vi "rqcSPI Write.vi"(9 "write data":bool, 11 "data in":u16) -> (1 "MOSI":bool, 2 "CLK":bool, 3 "CS":bool=TRUE)   [LabVIEW 2016]
uses:
  Custom Controls/rqcSPI Cluster.ctl
  Custom Controls/rqcSPI State.ctl
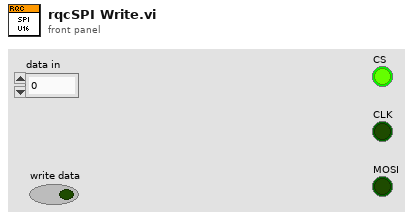
[diagram p1: front panel]
types:
  T1 = typedef "rqcSPI Cluster.ctl" = cluster{"state":T2, "bit's number":u8, "data":bool[], "CS":bool, "CLK":bool, "MOSI":bool}
  T2 = typedef "rqcSPI State.ctl" = enum16{"write", "idle"}
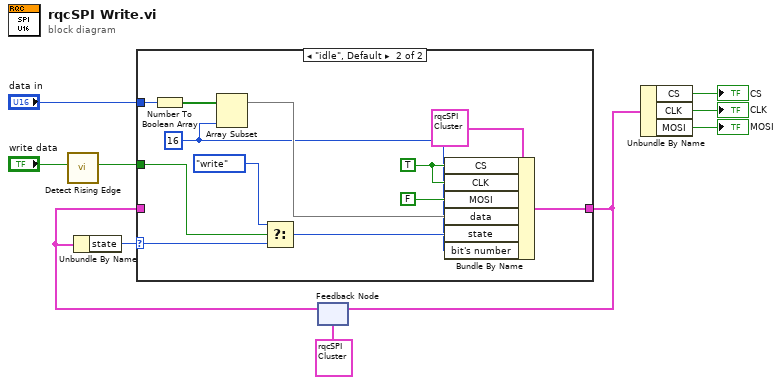
[diagram p0: block diagram]
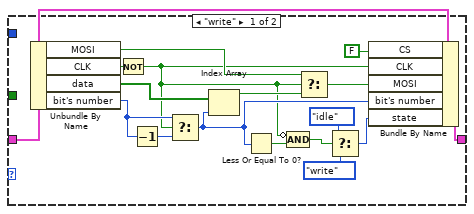
[diagram p2: hidden frame]
diagram:
  n1 = call <vilib>:"Detect Rising Edge.vi"("signal"="write data") -> ("edge detected"=w7:bool)  [unwired: 10 in]
  n2 = feedback #1(T1 {"state"=enum."idle", "bit's number"=16, "data"=[FALSE, FALSE, FALSE, FALSE, FALSE, FALSE, FALSE, FALSE, FALSE, FALSE, FALSE, FALSE, FALSE, FALSE, FALSE, FALSE], "CS"=TRUE, "CLK"=TRUE, "MOSI"=FALSE} ("rqcSPI Cluster")) -> (w6:T1)
  n3 = Unbundle By Name(w6) -> ("state"=w9:T2)
  n4 = case shown="\"idle\", Default" w9 {
    selector: w9 -> [_ w35]
    tunnel: w7 -> [_ w37]
    tunnel: w6 -> [w27 _]
    tunnel: "data in" -> [_ w38]
    tunnel: [w26 w33] -> w4
    frame "write" {
      n5 = Unbundle By Name(w27) -> ("MOSI"=w22:bool, "CLK"=w25:bool, "data"=w24:bool[], "bit's number"=w14:u8)
      n6 = Not(x=w25) -> (.not. x?=w12:bool)
      n7 = Decrement(x=w14) -> (x-1=w11:u8)
      n8 = Select(t=w14, s=w12, f=w11) -> (s? t:f=w15:u8)
      n9 = Index Array(array=w24, index=w15) -> (element=w23:bool)
      n10 = Less Or Equal To 0?(x=w15) -> (x <= 0?=w19:bool)
      n11 = Compound Arithmetic op=AND(invert w12, w19) -> (w13:bool)
      n12 = Select(t=w22, s=w12, f=w23) -> (s? t:f=w20:bool)
      n13 = Select(t=rqcSPI_State."idle", s=w13, f=rqcSPI_State."write" ("state")) -> (s? t:f=w16:T2)
      n14 = Bundle By Name(cluster=w27, "CS"=FALSE, "CLK"=w12, "MOSI"=w20, "bit's number"=w15, "state"=w16) -> (w26:T1)
    }
    frame "idle", Default {
      w31 = TRUE ("CS")
      w28 = u8 16 ("num of bit to write")
      n15 = Number To Boolean Array(number=w38) -> (Boolean array=w29:bool[])
      n16 = Array Subset(array=w29, length=w28) -> (w30:bool[])  [unwired: 1 in]
      n17 = Select(t=rqcSPI_State."write" ("state"), s=w37, f=w35) -> (s? t:f=w34:T2)
      n18 = Bundle By Name(cluster=T1 {"state"=enum."write", "bit's number"=0, "data"=[FALSE, FALSE, FALSE, FALSE, FALSE, FALSE, FALSE, FALSE, FALSE, FALSE, FALSE, FALSE, FALSE, FALSE, FALSE, FALSE], "CS"=FALSE, "CLK"=FALSE, "MOSI"=FALSE} ("rqcSPI Cluster"), "CS"=w31, "CLK"=w31, "MOSI"=FALSE, "data"=w30, "state"=w34, "bit's number"=w28) -> (w33:T1)
    }
  }
  n19 = feedback-in #1(w4) -> ()
  n20 = Unbundle By Name(w4) -> ("CS"=→"CS":bool, "CLK"=→"CLK":bool, "MOSI"=→"MOSI":bool)
